vi "InitImage.vi"() -> (3 "new picture":picture)   [LabVIEW 2020]
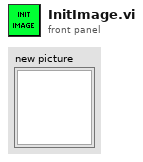
[diagram p1: front panel]
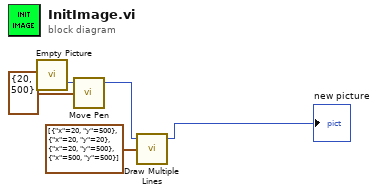
[diagram p0: block diagram]
diagram:
  n1 = call "Empty Picture"() -> ("empty picture"=w1:picture)
  n2 = call <vilib>:"Move Pen.vi"("new position"=cluster{"x":i16, "y":i16} {"x"=20, "y"=500}, "picture"=w1) -> ("new picture"=w5:picture)  [unwired: 3 in]
  n3 = call <vilib>:"Draw Multiple Lines.vi"("picture"=w5, "line endpoints"=cluster{"x":i16, "y":i16}[] [{"x"=20, "y"=500}, {"x"=20, "y"=20}, {"x"=20, "y"=500}, {"x"=500, "y"=500}]) -> ("new picture"=→"new picture":picture)  [unwired: 7 in]
